vi "ep_Speed Estimation for Single Motor (ICM).vi"(0 "signals":dbl[][](array[numeric]), 2 "reset? (F)":bool, 5 "fundamental frequency [Hz]":dbl format="%#_13g", 7 "nominal frequency":enum16{"50 Hz", "60 Hz"}(ring), 9 "nameplate speed":T1, 11 "error in (no error)":errorcluster, 12 "initial conditions":T2={"SVAF state"={"space vector amplitude"=0.0, "hilbert state"={"delay conditions"=[], "filter conditions"=[]}}, "zoom FFT state"={"phase state"=0.0, "zoom FFT state"={"zoom settings state"={"zoom"=0, "stop band attenuation"=enum."84 dB", "alias protect in final transition"=FALSE, "oversampling ratio"=0.0}, "SML Decimation Filter (complex input) state"={"decimation settings state"={"M"=0, "stop band attenuation"=enum."84 dB", "alias protect in transition band"=FALSE, "oversampling ratio"=0.0}, "counter for garbage samples state"=0, "sml_Parameter Setting for Zoom Factor state"={"filter length * interpolation state"=0, "interpolation state"=0, "comb filter order state"=0, "CFIR par state"={"h"=[], "M"=0, "N"=0}, "LFIR par state"={"h"=[], "M"=0, "N"=0}, "CIC Stages state"=0}, "aal_CIC (complex input) state"={"aal_cascaded moving average (complex input) state"={"states"=[], "circular buffers state"=[], "circular buffer counter state"=0}, "aal_moving average with decimation by order (complex input) state"={"residue result state"=0.0+0.0i, "processed data counter state"=0}}, "sml_Cascaded Decimation Filter (complex input) CFIR state"={"unprocessed data state"=[], "final conditions state"=[], "sml_M-1 Decimator with IC (complex input) state"={"coefficients in reverse order state"=[], "max index for coefficients state"=0}}, "sml_Cascaded Decimation Filter (complex input) LFIR state"={"unprocessed data state"=[], "final conditions state"=[], "sml_M-1 Decimator with IC (complex input) state"={"coefficients in reverse order state"=[], "max index for coefficients state"=0}}}, "ma_SML Data Packing (complex input) state"={"array getting packed state"=[], "last array processed state"=[], "index state"=0, "packing parameters state"={0, "size"=0}}}, "FFT{X} [Vrms]"=[]}, "speed state"={"speed [RPM]"=nan, "slip"=nan}, "speed estimation settings"={"% overlap"=0.0, "algorithm"=enum."3-phase signals"}, "filter information"={"coefficients"=[], "order"=0}, "zoom FFT settings"={"FFT settings"={"window"=0, "Window Size"=0, "FFT Size"=0, "%overlap"=0.0}, "zoom settings"={"zoom"=0, "stop band attenuation"=enum."84 dB", "alias protect in final transition"=FALSE, "oversampling ratio"=0.0}, "other settings"={"fmod"=0.0, "f0"=0.0, "df"=0.0, "oidx"=0, "olen"=0}, "iterations"=0, "max block size"=0, "fs"=0.0}, "last valid window"=0, "fund. frequency for averager"=[]} {"zoom FFT settings"."FFT settings"."window" items=["Rectangle"=0, "Hanning"=1, "Hamming"=2, "Blackman-Harris"=3, "Exact Blackman"=4, "Blackman"=5, "Flat Top"=6, "4 Term B-Harris "=7, "7 Term B-Harris"=8, "Low Sidelobe"=9, "Blackman Nuttall"=11, "Triangle"=30, "Bartlett-Hanning"=31, "Bohman"=32, "Parzen"=33, "Welch"=34, "Kaiser"=60, "Dolph-Chebyshev"=61, "Gaussian"=62]}) -> (3 "new speed available?":bool, 4 "speed [RPM]":dbl, 6 "slip":dbl, 13 "candidate speeds":cluster{"speed [RPM]":dbl, "slip":dbl}[](array[cluster]), 14 "final conditions":T2={"SVAF state"={"space vector amplitude"=0.0, "hilbert state"={"delay conditions"=[], "filter conditions"=[]}}, "zoom FFT state"={"phase state"=0.0, "zoom FFT state"={"zoom settings state"={"zoom"=0, "stop band attenuation"=enum."84 dB", "alias protect in final transition"=FALSE, "oversampling ratio"=0.0}, "SML Decimation Filter (complex input) state"={"decimation settings state"={"M"=0, "stop band attenuation"=enum."84 dB", "alias protect in transition band"=FALSE, "oversampling ratio"=0.0}, "counter for garbage samples state"=0, "sml_Parameter Setting for Zoom Factor state"={"filter length * interpolation state"=0, "interpolation state"=0, "comb filter order state"=0, "CFIR par state"={"h"=[], "M"=0, "N"=0}, "LFIR par state"={"h"=[], "M"=0, "N"=0}, "CIC Stages state"=0}, "aal_CIC (complex input) state"={"aal_cascaded moving average (complex input) state"={"states"=[], "circular buffers state"=[], "circular buffer counter state"=0}, "aal_moving average with decimation by order (complex input) state"={"residue result state"=0.0+0.0i, "processed data counter state"=0}}, "sml_Cascaded Decimation Filter (complex input) CFIR state"={"unprocessed data state"=[], "final conditions state"=[], "sml_M-1 Decimator with IC (complex input) state"={"coefficients in reverse order state"=[], "max index for coefficients state"=0}}, "sml_Cascaded Decimation Filter (complex input) LFIR state"={"unprocessed data state"=[], "final conditions state"=[], "sml_M-1 Decimator with IC (complex input) state"={"coefficients in reverse order state"=[], "max index for coefficients state"=0}}}, "ma_SML Data Packing (complex input) state"={"array getting packed state"=[], "last array processed state"=[], "index state"=0, "packing parameters state"={0, "size"=0}}}, "FFT{X} [Vrms]"=[]}, "speed state"={"speed [RPM]"=nan, "slip"=nan}, "speed estimation settings"={"% overlap"=0.0, "algorithm"=enum."3-phase signals"}, "filter information"={"coefficients"=[], "order"=0}, "zoom FFT settings"={"FFT settings"={"window"=0, "Window Size"=0, "FFT Size"=0, "%overlap"=0.0}, "zoom settings"={"zoom"=0, "stop band attenuation"=enum."84 dB", "alias protect in final transition"=FALSE, "oversampling ratio"=0.0}, "other settings"={"fmod"=0.0, "f0"=0.0, "df"=0.0, "oidx"=0, "olen"=0}, "iterations"=0, "max block size"=0, "fs"=0.0}, "last valid window"=0, "fund. frequency for averager"=[]} {"zoom FFT settings"."FFT settings"."window" items=["Rectangle"=0, "Hanning"=1, "Hamming"=2, "Blackman-Harris"=3, "Exact Blackman"=4, "Blackman"=5, "Flat Top"=6, "4 Term B-Harris "=7, "7 Term B-Harris"=8, "Low Sidelobe"=9, "Blackman Nuttall"=11, "Triangle"=30, "Bartlett-Hanning"=31, "Bohman"=32, "Parzen"=33, "Welch"=34, "Kaiser"=60, "Dolph-Chebyshev"=61, "Gaussian"=62]}, 15 "error out":errorcluster)   [LabVIEW 2017]
uses:
  <vilib>/addons/Electrical Power/Motor Monitoring/subVIs/ep_Initial Conditions for Speed Estimation.ctl
  <vilib>/addons/Electrical Power/Motor Monitoring/subVIs/ep_Demodulation Algorithm.ctl
  <vilib>/addons/Electrical Power/Motor Monitoring/subVIs/ep_Zoom FFT Settings.ctl
  <vilib>/addons/Electrical Power/Motor Monitoring/NI_EP_Motor Monitoring.lvlib
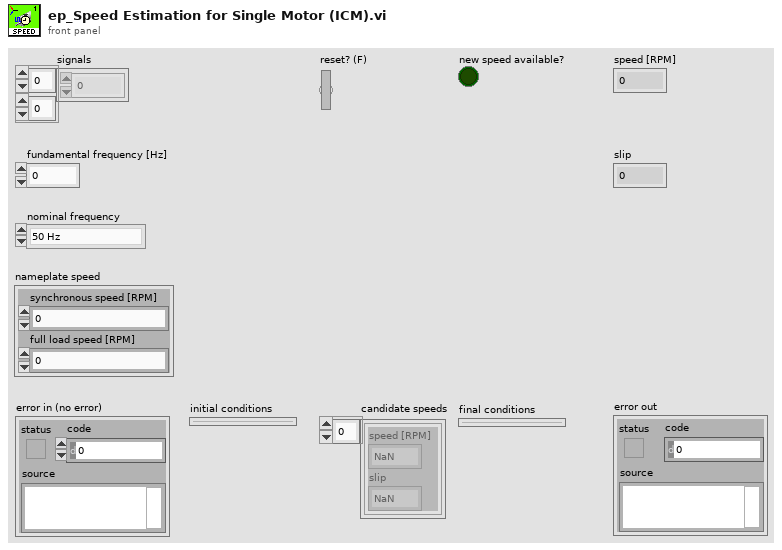
[diagram p1: front panel]
types:
  T1 = cluster{"synchronous speed [RPM]":dbl, "full load speed [RPM]":dbl}
  T2 = typedef "NI_EP_Motor Monitoring.lvlib/ep_Initial Conditions for Speed Estimation.ctl" = cluster{"SVAF state":cluster{"space vector amplitude":dbl, "hilbert state":cluster{"delay conditions":dbl[], "filter conditions":dbl[]}}, "zoom FFT state":cluster{"phase state":dbl, "zoom FFT state":cluster{"zoom settings state":cluster{"zoom":i32, "stop band attenuation":enum16{"84 dB", "96 dB", "120 dB"}, "alias protect in final transition":bool, "oversampling ratio":dbl}, "SML Decimation Filter (complex input) state":cluster{"decimation settings state":cluster{"M":i32, "stop band attenuation":enum16{"84 dB", "96 dB", "120 dB"}, "alias protect in transition band":bool, "oversampling ratio":dbl}, "counter for garbage samples state":i32, "sml_Parameter Setting for Zoom Factor state":cluster{"filter length * interpolation state":i32, "interpolation state":i32, "comb filter order state":i32, "CFIR par state":cluster{"h":dbl[], "M":i32, "N":i32}, "LFIR par state":cluster{"h":dbl[], "M":i32, "N":i32}, "CIC Stages state":i32}, "aal_CIC (complex input) state":cluster{"aal_cascaded moving average (complex input) state":cluster{"states":cdb[], "circular buffers state":cdb[][], "circular buffer counter state":i32}, "aal_moving average with decimation by order (complex input) state":cluster{"residue result state":cdb, "processed data counter state":i32}}, "sml_Cascaded Decimation Filter (complex input) CFIR state":cluster{"unprocessed data state":cdb[], "final conditions state":cdb[][], "sml_M-1 Decimator with IC (complex input) state":cluster{"coefficients in reverse order state":dbl[], "max index for coefficients state":i32}}, "sml_Cascaded Decimation Filter (complex input) LFIR state":cluster{"unprocessed data state":cdb[], "final conditions state":cdb[][], "sml_M-1 Decimator with IC (complex input) state":cluster{"coefficients in reverse order state":dbl[], "max index for coefficients state":i32}}}, "ma_SML Data Packing (complex input) state":cluster{"array getting packed state":cdb[], "last array processed state":cdb[], "index state":i32, "packing parameters state":cluster{i32, "size":i32}}}, "FFT{X} [Vrms]":cdb[]}, "speed state":cluster{"speed [RPM]":dbl, "slip":dbl}, "speed estimation settings":cluster{"% overlap":dbl, "algorithm":T3}, "filter information":cluster{"coefficients":dbl[], "order":i32}, "zoom FFT settings":T4, "last valid window":i32, "fund. frequency for averager":dbl[]}
  T3 = typedef "NI_EP_Motor Monitoring.lvlib/ep_Demodulation Algorithm.ctl" = enum16{"1-phase signal", "3-phase signals"}
  T4 = typedef "NI_EP_Motor Monitoring.lvlib/ep_Zoom FFT Settings.ctl" = cluster{"FFT settings":cluster{"window":u16, "Window Size":i32, "FFT Size":i32, "%overlap":dbl}, "zoom settings":cluster{"zoom":i32, "stop band attenuation":enum16{"84 dB", "96 dB", "120 dB"}, "alias protect in final transition":bool, "oversampling ratio":dbl}, "other settings":cluster{"fmod":dbl, "f0":dbl, "df":dbl, "oidx":i32, "olen":i32}, "iterations":i32, "max block size":i32, "fs":dbl}
  T5 = cluster{"space vector amplitude":dbl, "hilbert state":cluster{"delay conditions":dbl[], "filter conditions":dbl[]}}
  T6 = cluster{"phase state":dbl, "zoom FFT state":cluster{"zoom settings state":cluster{"zoom":i32, "stop band attenuation":enum16{"84 dB", "96 dB", "120 dB"}, "alias protect in final transition":bool, "oversampling ratio":dbl}, "SML Decimation Filter (complex input) state":cluster{"decimation settings state":cluster{"M":i32, "stop band attenuation":enum16{"84 dB", "96 dB", "120 dB"}, "alias protect in transition band":bool, "oversampling ratio":dbl}, "counter for garbage samples state":i32, "sml_Parameter Setting for Zoom Factor state":cluster{"filter length * interpolation state":i32, "interpolation state":i32, "comb filter order state":i32, "CFIR par state":cluster{"h":dbl[], "M":i32, "N":i32}, "LFIR par state":cluster{"h":dbl[], "M":i32, "N":i32}, "CIC Stages state":i32}, "aal_CIC (complex input) state":cluster{"aal_cascaded moving average (complex input) state":cluster{"states":cdb[], "circular buffers state":cdb[][], "circular buffer counter state":i32}, "aal_moving average with decimation by order (complex input) state":cluster{"residue result state":cdb, "processed data counter state":i32}}, "sml_Cascaded Decimation Filter (complex input) CFIR state":cluster{"unprocessed data state":cdb[], "final conditions state":cdb[][], "sml_M-1 Decimator with IC (complex input) state":cluster{"coefficients in reverse order state":dbl[], "max index for coefficients state":i32}}, "sml_Cascaded Decimation Filter (complex input) LFIR state":cluster{"unprocessed data state":cdb[], "final conditions state":cdb[][], "sml_M-1 Decimator with IC (complex input) state":cluster{"coefficients in reverse order state":dbl[], "max index for coefficients state":i32}}}, "ma_SML Data Packing (complex input) state":cluster{"array getting packed state":cdb[], "last array processed state":cdb[], "index state":i32, "packing parameters state":cluster{i32, "size":i32}}}, "FFT{X} [Vrms]":cdb[]}
  T7 = cluster{"maximum frequency [Hz]":dbl, "slip error allowance":dbl, "minimum points for peak search":dbl, "accuracy of fs":dbl, "difference?":bool, " fs harmonics order":i32, "fs forbidden range":dbl, "p3:p1 valid significance ratio":dbl, "ratio for significance weighting":dbl, "significance weighting":dbl}
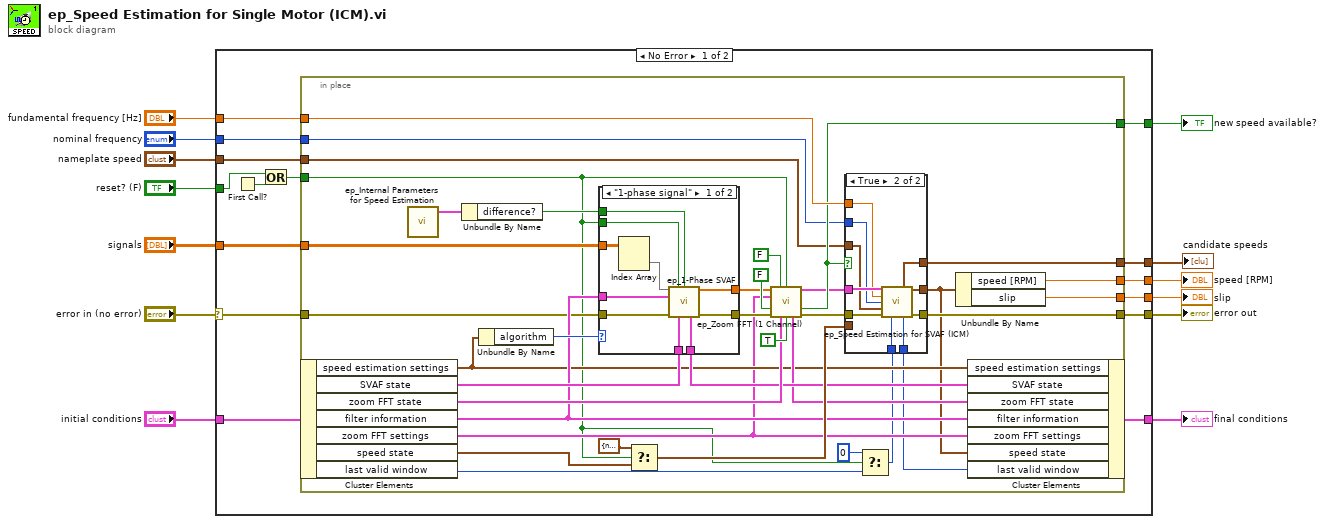
[diagram p0: block diagram]
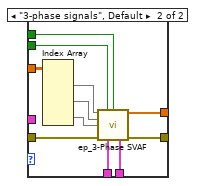
[diagram p3: hidden frame]
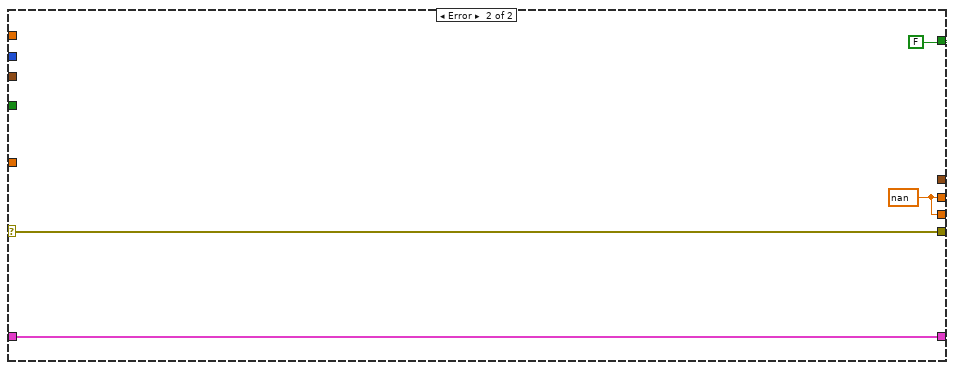
[diagram p4: hidden frame]
diagram:
  n1 = case shown="No Error" "error in (no error)" {
    selector: "error in (no error)" -> [w25 w102]
    tunnel: [w21 w102] -> w12
    tunnel: "reset? (F)" -> [w27 _]
    tunnel: "signals" -> [w26 _]
    tunnel: [w20 FALSE] -> w9
    tunnel: "nameplate speed" -> [w23 _]
    tunnel: "initial conditions" -> [w19 w100]
    tunnel: [w18 w100] -> w6
    tunnel: "fundamental frequency [Hz]" -> [w22 _]
    tunnel: "nominal frequency" -> [w17 _]
    tunnel: [w16 w99] -> w3
    tunnel: [w15 w99] -> w2
    tunnel: [w14 _] -> w1
    frame No Error {
      n2 = First Call?() -> (First Call?: T/F=w28:bool)
      n3 = Or(x=w27, y=w28) -> (x .or. y?=w24:bool)
      n4 = in-place {
        in-place-border: w26 -> [w62]
        in-place-border: w25 -> [w35]
        in-place-border: w24 -> [w31]
        in-place-border: w23 -> [w43]
        in-place-border: w22 -> [w57]
        in-place-border: [w55] -> w21
        in-place-border: [w54] -> w20
        in-place-border: w17 -> [w44]
        in-place-border: [w39] -> w16
        in-place-border: [w38] -> w15
        in-place-border: [w30] -> w14
        n5 = in-place-cluster #1(w19) -> ("speed estimation settings"=w46:cluster{"% overlap":dbl, "algorithm":T3}, "SVAF state"=w52:T5, "zoom FFT state"=w51:T6, "filter information"=w47:cluster{"coefficients":dbl[], "order":i32}, "zoom FFT settings"=w45:T4, "speed state"=w29:cluster{"speed [RPM]":dbl, "slip":dbl}, "last valid window"=w34:i32)
        n6 = call <vilib>:"ep_Internal Parameters for Speed Estimation.vi"() -> ("internal parameters for speed estimation"=w42:T7)  [unwired: 11 in]
        n7 = Unbundle By Name(w42) -> ("difference?"=w41:bool)
        n8 = Unbundle By Name(w46) -> ("algorithm"=w48:T3)
        n9 = case shown="\"1-phase signal\"" w48 {
          tunnel: w62 -> [w87 w98]
          tunnel: w31 -> [w84 w89]
          tunnel: w52 -> [w83 w94]
          tunnel: [w82 w93] -> w50
          tunnel: [w78 w92] -> w61
          tunnel: w35 -> [w80 w91]
          tunnel: [w81 w90] -> w60
          tunnel: w41 -> [w85 w88]
          tunnel: w47 -> [w79 _]
          frame "1-phase signal" {
            n10 = Index Array(array=w87) -> (element=w86:dbl[])  [unwired: 2 in]
            n11 = call <vilib>:"ep_1-Phase SVAF.vi"("signal"=w86, "reset? (F)"=w84, "difference? (T)"=w85, "filter information"=w79, "error in (no error)"=w80, "previous SVAF state"=w83) -> ("SVAF signal"=w78:dbl[], "next SVAF state"=w82:T5, "error out"=w81:errorcluster)  [unwired: 7 in]
          }
          frame "3-phase signals", Default {
            n12 = Index Array(array=w98) -> (element #1=w97:dbl[], element #2=w96:dbl[], element #3=w95:dbl[])  [unwired: 6 in]
            n13 = call <vilib>:"ep_3-Phase SVAF.vi"("phase A"=w97, "reset? (F)"=w89, "difference? (T)"=w88, "phase B"=w96, "phase C"=w95, "error in (no error)"=w91, "previous SVAF state"=w94) -> ("SVAF signal"=w92:dbl[], "next SVAF state"=w93:T5, "error out"=w90:errorcluster)  [unwired: 6 in]
          }
        }
        n14 = Select(t=cluster{"speed [RPM]":dbl, "slip":dbl} {"speed [RPM]"=nan, "slip"=nan}, s=w31, f=w29) -> (s? t:f=w58:cluster{"speed [RPM]":dbl, "slip":dbl})
        n15 = call <vilib>:"ep_Zoom FFT (1 Channel).vi"("signal"=w61, "phase output? (F)"=FALSE, "reset? (F)"=w31, "zoom FFT settings"=w45, "dB on? (T)"=FALSE, "error in (no error)"=w60, "zoom FFT state in"=w51, "demodulated? (F)"=TRUE) -> ("FFT magnitude"=w36:cluster{"f0":dbl, "df":dbl, "magnitude":dbl[]}, "spectrum ready?"=w54:bool, "zoom FFT state out"=w49:T6, "error out"=w56:errorcluster)  [unwired: 3 in, 1 out]
        n16 = Select(t=0, s=w31, f=w34) -> (s? t:f=w33:i32)
        n17 = case shown="True" w54 {
          tunnel: w58 -> [w67 _]
          tunnel: [w67 w72] -> w40
          tunnel: w36 -> [_ w77]
          tunnel: w43 -> [_ w71]
          tunnel: w57 -> [_ w76]
          tunnel: w56 -> [w66 w74]
          tunnel: [w66 w73] -> w55
          tunnel: w44 -> [_ w75]
          tunnel: w33 -> [w65 w70]
          tunnel: [w65 w69] -> w37
          tunnel: [_ w68] -> w30
          frame False {
          }
          frame True {
            n18 = call <vilib>:"ep_Speed Estimation for SVAF (ICM).vi"("SVAF spectrum"=w77, "fundamental frequency [Hz]"=w76, "nominal frequency"=w75, "nameplate speed"=w71, "error in (no error)"=w74, "last valid window"=w70) -> ("candidate speeds"=w68:cluster{"speed [RPM]":dbl, "slip":dbl}[], "speed data"=w72:cluster{"speed [RPM]":dbl, "slip":dbl}, "current valid window"=w69:i32, "error out"=w73:errorcluster)  [unwired: 6 in]
          }
        }
        n19 = Unbundle By Name(w40) -> ("speed [RPM]"=w39:dbl, "slip"=w38:dbl)
        n20 = in-place-cluster #1("speed estimation settings"=w46, "SVAF state"=w50, "zoom FFT state"=w49, "filter information"=w47, "zoom FFT settings"=w45, "speed state"=w40, "last valid window"=w37) -> (w18:T2)
      }
    }
    frame Error {
      w99 = nan ("speed [RPM]")
    }
  }
  "error out" <- w12
  "new speed available?" <- w9
  "final conditions" <- w6
  "speed [RPM]" <- w3
  "slip" <- w2
  "candidate speeds" <- w1
